vi "Tell Reply.vi"(4 "Priority":bool, 10 "Msg":refnum<class "Msg.lvclass">, 11 "Base Actor in":refnum<class "Base Actor.lvclass">) -> (0 "Error out":errorcluster)   [LabVIEW 2025, in "jettl.lvlib" / "Actor.lvlib" / "Base Actor.lvclass"]
uses:
  Base Actor.lvclass
  Base Actor.lvclass/Base Actor.ctl
  Teller/Teller/Teller.lvclass
  Error/Error.lvlib
  Msg/Msg.lvclass
  Attributes/Attributes/Attributes.lvclass
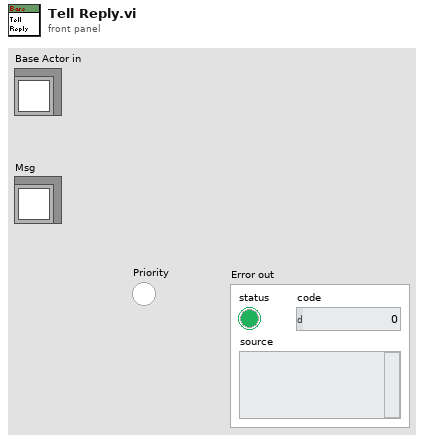
[diagram p1: front panel]
types:
  T1 = typedef "jettl.lvlib/Actor.lvlib/Relation.ctl" = enum16{"Self", "Creator", "Created"}
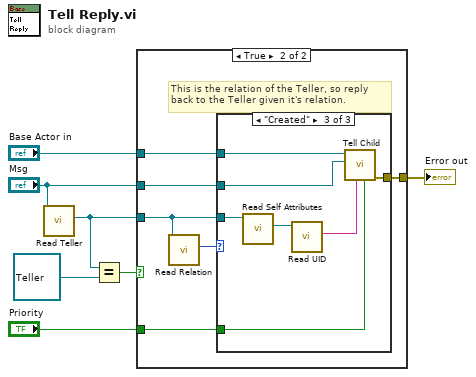
[diagram p0: block diagram]
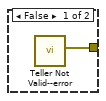
[diagram p2: hidden frame]
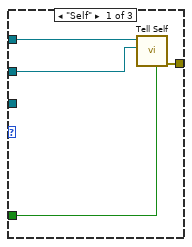
[diagram p3: hidden frame]
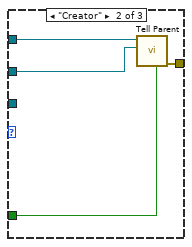
[diagram p4: hidden frame]
diagram:
  n1 = call-dynamic "Read Teller.vi"("Msg in"="Msg") -> ("Teller"=w1:refnum<class "Teller.lvclass">)  [unwired: 10 in]
  n2 = Equal?(x=w1, y=refnum<class "Teller.lvclass"> refnum ("Sender")) -> (x = y?=w4:bool)
  n3 = case shown="True" w4 {
    tunnel: "Base Actor in" -> [_ w14]
    tunnel: "Msg" -> [_ w13]
    tunnel: "Priority" -> [_ w12]
    tunnel: w1 -> [_ w11]
    tunnel: [w8 w9] -> w5
    frame False {
      n4 = call "Teller Not Valid--error.vi"() -> ("Error"=w8:errorcluster)  [unwired: 11 in]
    }
    frame True {
      # "This is the relation of the Teller, so reply back to the Teller given it's relation."
      n5 = call-dynamic "Read Relation.vi"("Teller in"=w11) -> ("Relation"=w10:T1)  [unwired: 10 in]
      n6 = case shown="\"Created\"" w10 {
        tunnel: w14 -> [w18 w22 w29]
        tunnel: w13 -> [w17 w21 w28]
        tunnel: w12 -> [w15 w19 w23]
        tunnel: w11 -> [_ _ w27]
        tunnel: [w16 w20 w25] -> w9
        frame "Self" {
          n7 = call-dynamic "Tell Self.vi"("Priority"=w15, "Msg"=w17, "Base Actor in"=w18) -> ("Error out"=w16:errorcluster)  [unwired: 8 in]
        }
        frame "Creator" {
          n8 = call-dynamic "Tell Parent.vi"("Priority"=w19, "Msg"=w21, "Base Actor in"=w22) -> ("Error out"=w20:errorcluster)  [unwired: 8 in]
        }
        frame "Created" {
          n9 = call-dynamic "Read Self Attributes.vi"("Teller in"=w27) -> ("Self Attributes"=w26:refnum<class "Attributes.lvclass">)  [unwired: 10 in]
          n10 = call-dynamic "Read UID.vi"("Attributes in"=w26) -> ("UID"=w24:string)  [unwired: 10 in]
          n11 = call-dynamic "Tell Child.vi"("Priority"=w23, "UID"=w24, "Msg"=w28, "Base Actor in"=w29) -> ("Error out"=w25:errorcluster)  [unwired: 7 in]
        }
      }
    }
  }
  "Error out" <- w5
